vi "Close Refnum.vi"(8 "Error In":errorcluster, 11 "Divide In":refnum<class "Divide.lvclass">) -> (0 "Error Out":errorcluster, 3 "Divide Out":refnum<class "Divide.lvclass">)   [LabVIEW 2021, in "Calculator.lvlib" / "Divide.lvclass"]
doc: "This VI is a overriding method which closes the subpanel reference."
uses:
  Divide.lvclass
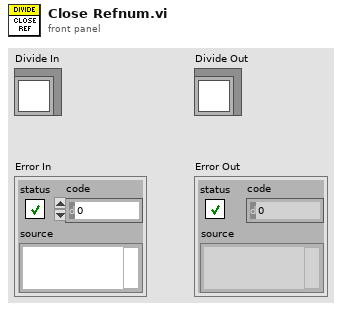
[diagram p1: front panel]
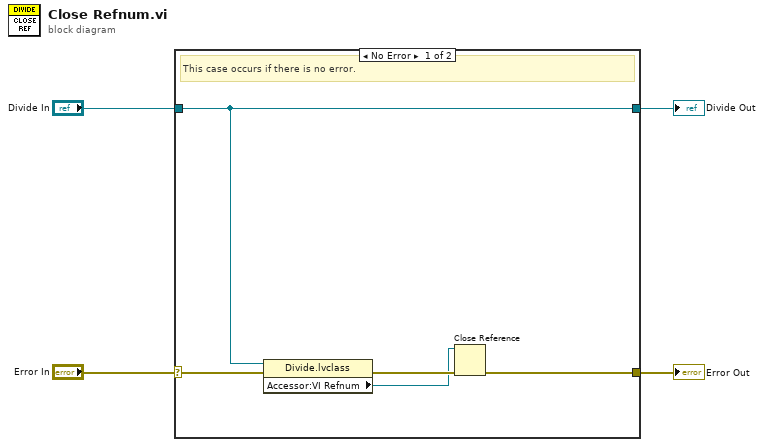
[diagram p0: block diagram]
diagram:
  n1 = case shown="No Error" "Error In" {
    selector: "Error In" -> [w9 w11]
    tunnel: [w6 w11] -> w3
    tunnel: [w7 w10] -> w1
    tunnel: "Divide In" -> [w7 w10]
    frame No Error {
      # "This case occurs if there is no error."
      n2 = property class="Divide.lvclass"(reference=w7, error in=w9) -> (error out=w8:errorcluster, "Accessor:VI Refnum"=w5:refnum<vi>)  [unwired: 1 out]
      n3 = Close Reference(reference=w5, error in (no error)=w8) -> (error out=w6:errorcluster)
    }
    frame Error {
      # "This case occurs if there is no error."
    }
  }
  "Error Out" <- w3
  "Divide Out" <- w1
